vi "WinCI Provider Supports Functionality.vi"(8 "error in (no error)":errorcluster, 10 "functionality":T1) -> (0 "error out":errorcluster, 2 "provider supports?":bool)   [LabVIEW 2017, in "NI_SCC_WinCI.lvlib"]
uses:
  <vilib>/SourceControl/Providers/WinCI/NI_SCC_WinCI.lvlib
  <vilib>/SourceControl/sccapi/SCCAPI SCC Provider Functionality.ctl
  <vilib>/SourceControl/Providers/WinCI/WinCI Interface Command.ctl
  <vilib>/SourceControl/Providers/WinCI/WinCI Interface Functionality.ctl
  <vilib>/SourceControl/sccapi/NI_SCC.lvlib
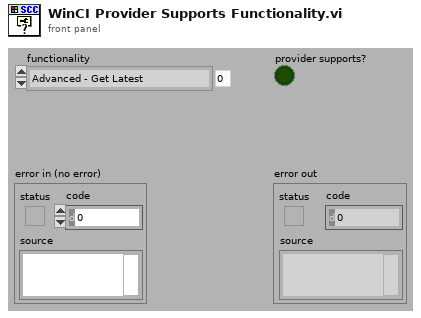
[diagram p1: front panel]
types:
  T1 = typedef "NI_SCC.lvlib/SCCAPI SCC Provider Functionality.ctl" = enum16{"Advanced - Get Latest", "Advanced - CheckOut", "Advanced - CheckIn", "Advanced - UndoCheckOut", "Advanced - Add", "Advanced - Remove", "Advanced - FileCompare", "Advanced - FileHistory", "Advanced - FileProperties", "Advanced - ConfigOptions", "Run SCC", "Configure Project", "Comment on CheckOut", "Comment on CheckIn", "Comment on Add", "Comment on Remove", "Keep Checked Out", "Get File Copy", "Multifile History"}
  T2 = typedef "NI_SCC_WinCI.lvlib/WinCI Interface Command.ctl" = i32
  T3 = typedef "NI_SCC_WinCI.lvlib/WinCI Interface Functionality.ctl" = i32
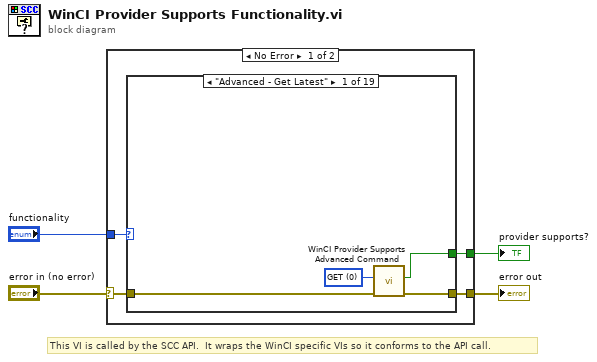
[diagram p0: block diagram]
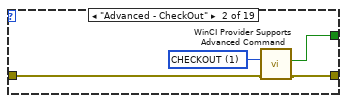
[diagram p2: hidden frame]
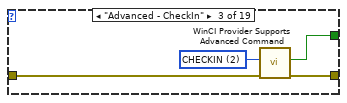
[diagram p3: hidden frame]
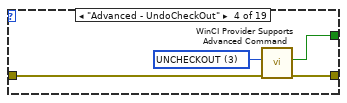
[diagram p4: hidden frame]
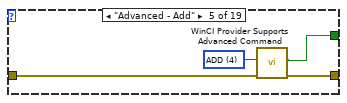
[diagram p5: hidden frame]
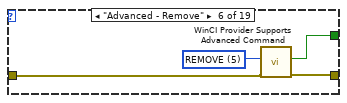
[diagram p6: hidden frame]
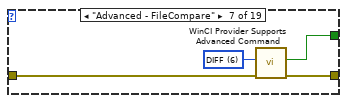
[diagram p7: hidden frame]
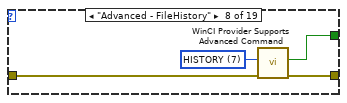
[diagram p8: hidden frame]
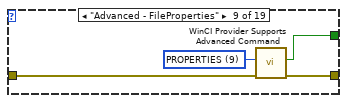
[diagram p9: hidden frame]
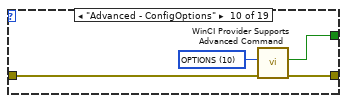
[diagram p10: hidden frame]
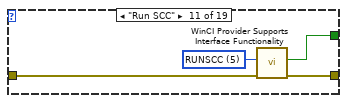
[diagram p11: hidden frame]
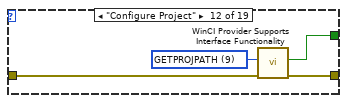
[diagram p12: hidden frame]
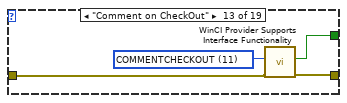
[diagram p13: hidden frame]
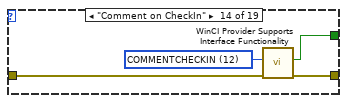
[diagram p14: hidden frame]
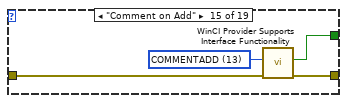
[diagram p15: hidden frame]
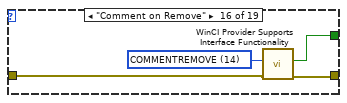
[diagram p16: hidden frame]
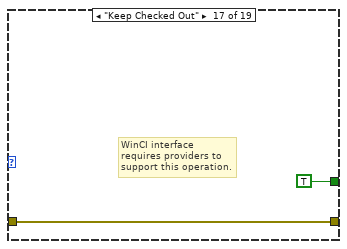
[diagram p17: hidden frame]
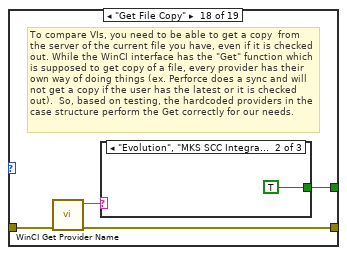
[diagram p18: hidden frame]
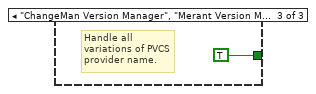
[diagram p20: hidden frame]
diagram:
  # "This VI is called by the SCC API.  It wraps the WinCI specific VIs so it conforms to the API call."
  n1 = case shown="No Error" "error in (no error)" {
    selector: "error in (no error)" -> [w8 w85]
    tunnel: [w6 w85] -> w3
    tunnel: [w5 _] -> w2
    tunnel: "functionality" -> [w7 _]
    frame No Error {
      n2 = case shown="\"Advanced - Get Latest\"" w7 {
        tunnel: w8 -> [w11 w15 w19 w24 w26 w29 w36 w39 w43 w46 w50 w54 w57 w61 w67 w71 w74 w75 w81]
        tunnel: [w10 w16 w20 w23 w27 w30 w35 w40 w44 w47 w49 w53 w58 w62 w68 w72 w74 w76 w82] -> w6
        tunnel: [w9 w13 w17 w22 w28 w31 w34 w38 w42 w48 w52 w56 w59 w63 w66 w70 TRUE ("provider supports?") w78 w83] -> w5
        frame "Advanced - Get Latest" {
          w12 = T2 0 items=["GET", "CHECKOUT", "CHECKIN", "UNCHECKOUT", "ADD", "REMOVE", "DIFF", "HISTORY", "RENAME", "PROPERTIES", "OPTIONS"] ("interface command")
          n3 = call <vilib>:"WinCI Provider Supports Advanced Command.vi"("error in (no error)"=w11, "interface command"=w12) -> ("error out"=w10:errorcluster, "provider supports?"=w9:bool)  [unwired: 8 out]
        }
        frame "Advanced - CheckOut" {
          w14 = T2 1 items=["GET", "CHECKOUT", "CHECKIN", "UNCHECKOUT", "ADD", "REMOVE", "DIFF", "HISTORY", "RENAME", "PROPERTIES", "OPTIONS"] ("interface command")
          n4 = call <vilib>:"WinCI Provider Supports Advanced Command.vi"("error in (no error)"=w15, "interface command"=w14) -> ("error out"=w16:errorcluster, "provider supports?"=w13:bool)  [unwired: 8 out]
        }
        frame "Advanced - CheckIn" {
          w18 = T2 2 items=["GET", "CHECKOUT", "CHECKIN", "UNCHECKOUT", "ADD", "REMOVE", "DIFF", "HISTORY", "RENAME", "PROPERTIES", "OPTIONS"] ("interface command")
          n5 = call <vilib>:"WinCI Provider Supports Advanced Command.vi"("error in (no error)"=w19, "interface command"=w18) -> ("error out"=w20:errorcluster, "provider supports?"=w17:bool)  [unwired: 8 out]
        }
        frame "Advanced - UndoCheckOut" {
          w21 = T2 3 items=["GET", "CHECKOUT", "CHECKIN", "UNCHECKOUT", "ADD", "REMOVE", "DIFF", "HISTORY", "RENAME", "PROPERTIES", "OPTIONS"] ("interface command")
          n6 = call <vilib>:"WinCI Provider Supports Advanced Command.vi"("error in (no error)"=w24, "interface command"=w21) -> ("error out"=w23:errorcluster, "provider supports?"=w22:bool)  [unwired: 8 out]
        }
        frame "Advanced - Add" {
          w25 = T2 4 items=["GET", "CHECKOUT", "CHECKIN", "UNCHECKOUT", "ADD", "REMOVE", "DIFF", "HISTORY", "RENAME", "PROPERTIES", "OPTIONS"] ("interface command")
          n7 = call <vilib>:"WinCI Provider Supports Advanced Command.vi"("error in (no error)"=w26, "interface command"=w25) -> ("error out"=w27:errorcluster, "provider supports?"=w28:bool)  [unwired: 8 out]
        }
        frame "Advanced - Remove" {
          w32 = T2 5 items=["GET", "CHECKOUT", "CHECKIN", "UNCHECKOUT", "ADD", "REMOVE", "DIFF", "HISTORY", "RENAME", "PROPERTIES", "OPTIONS"] ("interface command")
          n8 = call <vilib>:"WinCI Provider Supports Advanced Command.vi"("error in (no error)"=w29, "interface command"=w32) -> ("error out"=w30:errorcluster, "provider supports?"=w31:bool)  [unwired: 8 out]
        }
        frame "Advanced - FileCompare" {
          w33 = T2 6 items=["GET", "CHECKOUT", "CHECKIN", "UNCHECKOUT", "ADD", "REMOVE", "DIFF", "HISTORY", "RENAME", "PROPERTIES", "OPTIONS"] ("interface command")
          n9 = call <vilib>:"WinCI Provider Supports Advanced Command.vi"("error in (no error)"=w36, "interface command"=w33) -> ("error out"=w35:errorcluster, "provider supports?"=w34:bool)  [unwired: 8 out]
        }
        frame "Advanced - FileHistory" {
          w37 = T2 7 items=["GET", "CHECKOUT", "CHECKIN", "UNCHECKOUT", "ADD", "REMOVE", "DIFF", "HISTORY", "RENAME", "PROPERTIES", "OPTIONS"] ("interface command")
          n10 = call <vilib>:"WinCI Provider Supports Advanced Command.vi"("error in (no error)"=w39, "interface command"=w37) -> ("error out"=w40:errorcluster, "provider supports?"=w38:bool)  [unwired: 8 out]
        }
        frame "Advanced - FileProperties" {
          w41 = T2 9 items=["GET", "CHECKOUT", "CHECKIN", "UNCHECKOUT", "ADD", "REMOVE", "DIFF", "HISTORY", "RENAME", "PROPERTIES", "OPTIONS"] ("interface command")
          n11 = call <vilib>:"WinCI Provider Supports Advanced Command.vi"("error in (no error)"=w43, "interface command"=w41) -> ("error out"=w44:errorcluster, "provider supports?"=w42:bool)  [unwired: 8 out]
        }
        frame "Advanced - ConfigOptions" {
          w45 = T2 10 items=["GET", "CHECKOUT", "CHECKIN", "UNCHECKOUT", "ADD", "REMOVE", "DIFF", "HISTORY", "RENAME", "PROPERTIES", "OPTIONS"] ("interface command")
          n12 = call <vilib>:"WinCI Provider Supports Advanced Command.vi"("error in (no error)"=w46, "interface command"=w45) -> ("error out"=w47:errorcluster, "provider supports?"=w48:bool)  [unwired: 8 out]
        }
        frame "Run SCC" {
          w51 = T3 5 items=["REMOVE", "RENAME", "DIFF", "HISTORY", "PROPERTIES", "RUNSCC", "GETCOMMANDOPTIONS", "QUERYINFO", "GETEVENTS", "GETPROJPATH", "ADDFROMSCC", "COMMENTCHECKOUT", "COMMENTCHECKIN", "COMMENTADD", "COMMENTREMOVE", "TEXTOUT", "ADD_STORELATEST", "HISTORY_MULTIFILE", "IGNORECASE", "IGNORESPACE", "POPULATELIST", "COMMENTPROJECT", "DIFFALWAYS", "GET_NOUI", "REENTRANT"] ("interface functionality")
          n13 = call <vilib>:"WinCI Provider Supports Interface Functionality.vi"("error in (no error)"=w50, "interface functionality"=w51) -> ("error out"=w49:errorcluster, "provider supports?"=w52:bool)  [unwired: 8 out]
        }
        frame "Configure Project" {
          w55 = T3 9 items=["REMOVE", "RENAME", "DIFF", "HISTORY", "PROPERTIES", "RUNSCC", "GETCOMMANDOPTIONS", "QUERYINFO", "GETEVENTS", "GETPROJPATH", "ADDFROMSCC", "COMMENTCHECKOUT", "COMMENTCHECKIN", "COMMENTADD", "COMMENTREMOVE", "TEXTOUT", "ADD_STORELATEST", "HISTORY_MULTIFILE", "IGNORECASE", "IGNORESPACE", "POPULATELIST", "COMMENTPROJECT", "DIFFALWAYS", "GET_NOUI", "REENTRANT"] ("interface functionality")
          n14 = call <vilib>:"WinCI Provider Supports Interface Functionality.vi"("error in (no error)"=w54, "interface functionality"=w55) -> ("error out"=w53:errorcluster, "provider supports?"=w56:bool)  [unwired: 8 out]
        }
        frame "Comment on CheckOut" {
          w60 = T3 11 items=["REMOVE", "RENAME", "DIFF", "HISTORY", "PROPERTIES", "RUNSCC", "GETCOMMANDOPTIONS", "QUERYINFO", "GETEVENTS", "GETPROJPATH", "ADDFROMSCC", "COMMENTCHECKOUT", "COMMENTCHECKIN", "COMMENTADD", "COMMENTREMOVE", "TEXTOUT", "ADD_STORELATEST", "HISTORY_MULTIFILE", "IGNORECASE", "IGNORESPACE", "POPULATELIST", "COMMENTPROJECT", "DIFFALWAYS", "GET_NOUI", "REENTRANT"] ("interface functionality")
          n15 = call <vilib>:"WinCI Provider Supports Interface Functionality.vi"("error in (no error)"=w57, "interface functionality"=w60) -> ("error out"=w58:errorcluster, "provider supports?"=w59:bool)  [unwired: 8 out]
        }
        frame "Comment on CheckIn" {
          w64 = T3 12 items=["REMOVE", "RENAME", "DIFF", "HISTORY", "PROPERTIES", "RUNSCC", "GETCOMMANDOPTIONS", "QUERYINFO", "GETEVENTS", "GETPROJPATH", "ADDFROMSCC", "COMMENTCHECKOUT", "COMMENTCHECKIN", "COMMENTADD", "COMMENTREMOVE", "TEXTOUT", "ADD_STORELATEST", "HISTORY_MULTIFILE", "IGNORECASE", "IGNORESPACE", "POPULATELIST", "COMMENTPROJECT", "DIFFALWAYS", "GET_NOUI", "REENTRANT"] ("interface functionality")
          n16 = call <vilib>:"WinCI Provider Supports Interface Functionality.vi"("error in (no error)"=w61, "interface functionality"=w64) -> ("error out"=w62:errorcluster, "provider supports?"=w63:bool)  [unwired: 8 out]
        }
        frame "Comment on Add" {
          w65 = T3 13 items=["REMOVE", "RENAME", "DIFF", "HISTORY", "PROPERTIES", "RUNSCC", "GETCOMMANDOPTIONS", "QUERYINFO", "GETEVENTS", "GETPROJPATH", "ADDFROMSCC", "COMMENTCHECKOUT", "COMMENTCHECKIN", "COMMENTADD", "COMMENTREMOVE", "TEXTOUT", "ADD_STORELATEST", "HISTORY_MULTIFILE", "IGNORECASE", "IGNORESPACE", "POPULATELIST", "COMMENTPROJECT", "DIFFALWAYS", "GET_NOUI", "REENTRANT"] ("interface functionality")
          n17 = call <vilib>:"WinCI Provider Supports Interface Functionality.vi"("error in (no error)"=w67, "interface functionality"=w65) -> ("error out"=w68:errorcluster, "provider supports?"=w66:bool)  [unwired: 8 out]
        }
        frame "Comment on Remove" {
          w69 = T3 14 items=["REMOVE", "RENAME", "DIFF", "HISTORY", "PROPERTIES", "RUNSCC", "GETCOMMANDOPTIONS", "QUERYINFO", "GETEVENTS", "GETPROJPATH", "ADDFROMSCC", "COMMENTCHECKOUT", "COMMENTCHECKIN", "COMMENTADD", "COMMENTREMOVE", "TEXTOUT", "ADD_STORELATEST", "HISTORY_MULTIFILE", "IGNORECASE", "IGNORESPACE", "POPULATELIST", "COMMENTPROJECT", "DIFFALWAYS", "GET_NOUI", "REENTRANT"] ("interface functionality")
          n18 = call <vilib>:"WinCI Provider Supports Interface Functionality.vi"("error in (no error)"=w71, "interface functionality"=w69) -> ("error out"=w72:errorcluster, "provider supports?"=w70:bool)  [unwired: 8 out]
        }
        frame "Keep Checked Out" {
          # "WinCI interface requires providers to support this operation."
        }
        frame "Get File Copy" {
          # "To compare VIs, you need to be able to get a copy  from the server of the current file you have, even if it is checked out. While the WinCI interface has the \"Get\" function which is supposed to get copy of a file, every provider has their own way of doing things (ex. Perforce does a sync and will not get a copy if the user has the latest or it is checked out).  So, based on testing, the hardcoded providers in the case structure perform the Get correctly for our needs."
          n19 = call <vilib>:"WinCI Get Provider Name.vi"("error in (no error)"=w75) -> ("error out"=w76:errorcluster, "provider name"=w77:string)  [unwired: 9 out]
          n20 = case shown="\"Evolution\", \"MKS SCC Integration\", \"Microsoft Visual SourceSafe\", \"PushOk CVS Proxy\", \"PushOk SVN Proxy\", \"StarTeam\", \"Surround SCM\", \"Team Foundation Server MSSCCI Provider\"" w77 {
            tunnel: [_ TRUE ("provider supports?") TRUE ("provider supports?")] -> w78
            frame Default {
              # "Empirically determined that Clearcase, Perforce SCM, and CM Synergy do not support getting a file copy."
            }
            frame "Evolution", "MKS SCC Integration", "Microsoft Visual SourceSafe", "PushOk CVS Proxy", "PushOk SVN Proxy", "StarTeam", "Surround SCM", "Team Foundation Server MSSCCI Provider" {
            }
            frame "ChangeMan Version Manager", "Merant Version Manager", "PVCS" {
              # "Handle all variations of PVCS provider name."
            }
          }
        }
        frame "Multifile History" {
          w84 = T3 17 items=["REMOVE", "RENAME", "DIFF", "HISTORY", "PROPERTIES", "RUNSCC", "GETCOMMANDOPTIONS", "QUERYINFO", "GETEVENTS", "GETPROJPATH", "ADDFROMSCC", "COMMENTCHECKOUT", "COMMENTCHECKIN", "COMMENTADD", "COMMENTREMOVE", "TEXTOUT", "ADD_STORELATEST", "HISTORY_MULTIFILE", "IGNORECASE", "IGNORESPACE", "POPULATELIST", "COMMENTPROJECT", "DIFFALWAYS", "GET_NOUI", "REENTRANT"] ("interface functionality")
          n21 = call <vilib>:"WinCI Provider Supports Interface Functionality.vi"("error in (no error)"=w81, "interface functionality"=w84) -> ("error out"=w82:errorcluster, "provider supports?"=w83:bool)  [unwired: 8 out]
        }
      }
    }
    frame Error {
    }
  }
  "error out" <- w3
  "provider supports?" <- w2
